vi "Read Loops.vi"(8 "error in (no error)":errorcluster, 11 "Measurement3D in":refnum<class "Measurement3D.lvclass">) -> (0 "error out":errorcluster, 1 "Outer Loop":T1, 2 "Inner Loop":T2, 3 "Measurement3D out":refnum<class "Measurement3D.lvclass">)   [LabVIEW 2014, in "Measurement3D.lvclass"]
uses:
  Measurement3D.lvclass
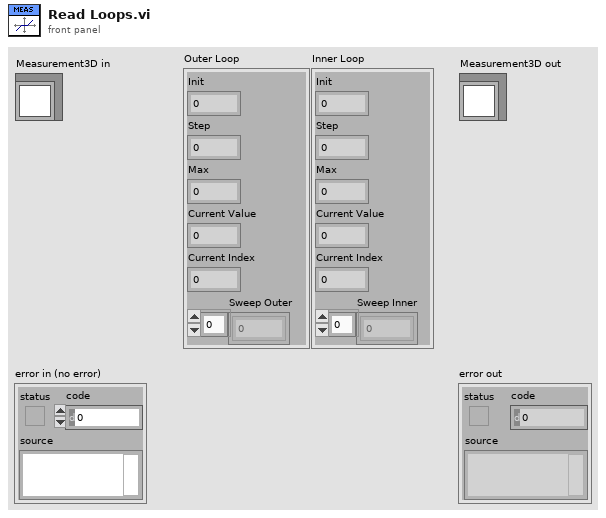
[diagram p1: front panel]
types:
  T1 = cluster{"Init":dbl, "Step":dbl, "Max":dbl, "Current Value":dbl, "Current Index":dbl, "Sweep Outer":dbl[]}
  T2 = cluster{"Init":dbl, "Step":dbl, "Max":dbl, "Current Value":dbl, "Current Index":dbl, "Sweep Inner":dbl[]}
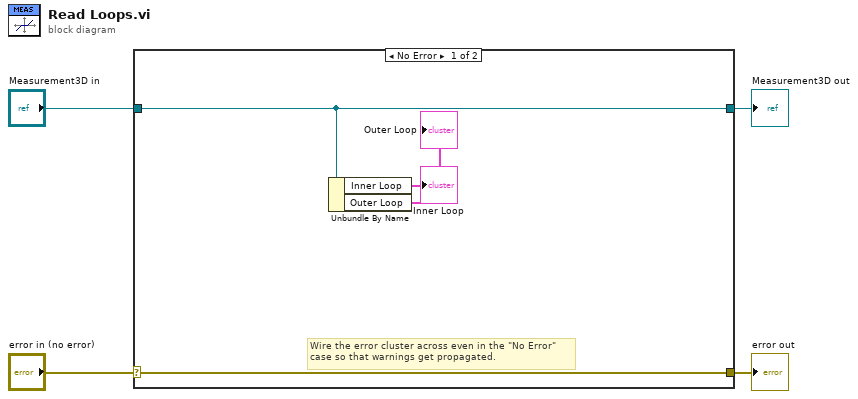
[diagram p0: block diagram]
diagram:
  n1 = case shown="No Error" "error in (no error)" {
    selector: "error in (no error)" -> [w8 w10]
    tunnel: [w8 w10] -> w3
    tunnel: [w7 w9] -> w1
    tunnel: "Measurement3D in" -> [w7 w9]
    frame No Error {
      # "Wire the error cluster across even in the \"No Error\"\ncase so that warnings get propagated."
      n2 = Unbundle By Name(w7) -> ("Inner Loop"=→"Inner Loop":T2, "Outer Loop"=→"Outer Loop":T1)
    }
    frame Error {
    }
  }
  "error out" <- w3
  "Measurement3D out" <- w1
